vi "Init.vi"(8 "error in (no error)":errorcluster) -> (0 "error out":errorcluster, 3 "Mock Data Listener Out":refnum<class "Mock Data Listener.lvclass">)   [LabVIEW 2020, in "Mock Data Listener.lvclass"]
uses:
  Mock Data Listener.lvclass
  Mock Data Listener.lvclass/Mock Data Listener.ctl
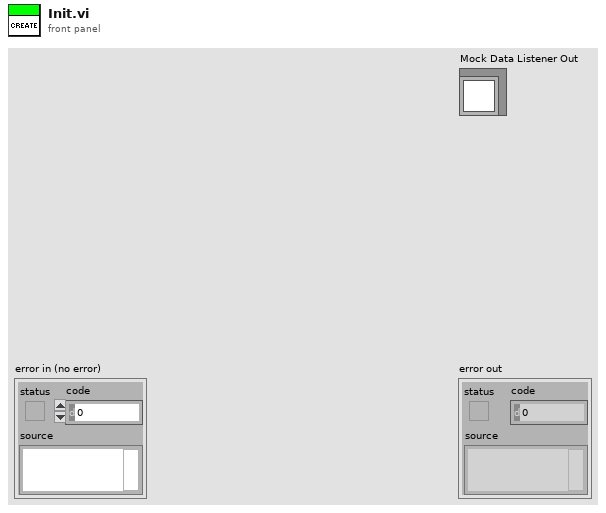
[diagram p1: front panel]
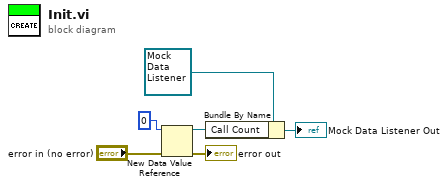
[diagram p0: block diagram]
diagram:
  n1 = New Data Value Reference(data value=0, error in="error in (no error)") -> (data value reference=w3:refnum<data-value>, error out=→"error out":errorcluster)
  n2 = Bundle By Name(cluster=refnum<class "Mock Data Listener.lvclass"> refnum ("Mock Data Listener in"), "Call Count"=w3) -> (→"Mock Data Listener Out":refnum<class "Mock Data Listener.lvclass">)
